vi "GEOM_GUI_trans_geom.vi"(10 "amps in":T1={"number"=0, "type"=0, "rotated"=0, "fliped"=0, "FPAcoord"={"xstart"=1, "ystart"=1}, "Physical_size"={"columns"=0, "rows"=0}, "predata"={"columns"=0, "rows"=0}, "postdata"={"columns"=0, "rows"=0}, "Req ROIs"=[], "Corr ROI"=[], "Detnumber"=0, "ampID"="", "discard"=0} {"fliped" items=["none", "horizontal", "vertical"]; "type" items=["LL", "LR", "UL", "UR"]}) -> (1 "amp direction":string, 2 "amps out":T1={"number"=0, "type"=0, "rotated"=0, "fliped"=0, "FPAcoord"={"xstart"=1, "ystart"=1}, "Physical_size"={"columns"=0, "rows"=0}, "predata"={"columns"=0, "rows"=0}, "postdata"={"columns"=0, "rows"=0}, "Req ROIs"=[], "Corr ROI"=[], "Detnumber"=0, "ampID"="", "discard"=0} {"fliped" items=["none", "horizontal", "vertical"]; "type" items=["LL", "LR", "UL", "UR"]})   [LabVIEW 2016]
uses:
  private/vis/GEOM_Amplifier.ctl
  private/vis/GEOM_AmpType.ctl
  private/vis/GEOM_ROI.ctl
  private/vis/GEOM_Coords.ctl
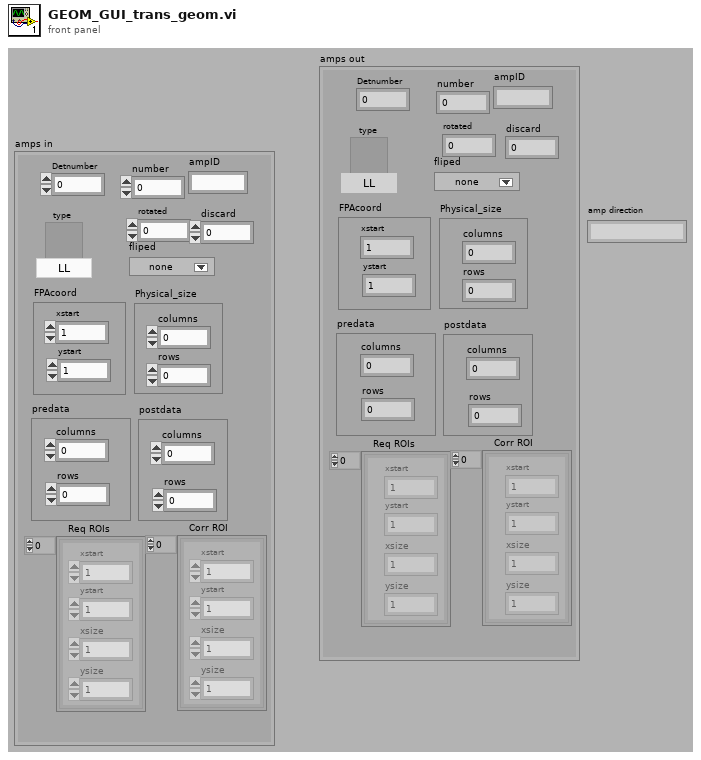
[diagram p1: front panel]
types:
  T1 = typedef "GEOM_Amplifier.ctl" = cluster{"number":i32, "type":T2, "rotated":i16, "fliped":u16, "FPAcoord":cluster{"xstart":i32, "ystart":i32}, "Physical_size":cluster{"columns":i32, "rows":i32}, "predata":cluster{"columns":i32, "rows":i32}, "postdata":cluster{"columns":i32, "rows":i32}, "Req ROIs":T3, "Corr ROI":T3, "Detnumber":i32, "ampID":string, "discard":i32}
  T2 = typedef "GEOM_AmpType.ctl" = u16
  T3 = typedef "GEOM_ROI.ctl" = T4[]
  T4 = typedef "GEOM_Coords.ctl" = cluster{"xstart":u32, "ystart":u32, "xsize":u32, "ysize":u32}
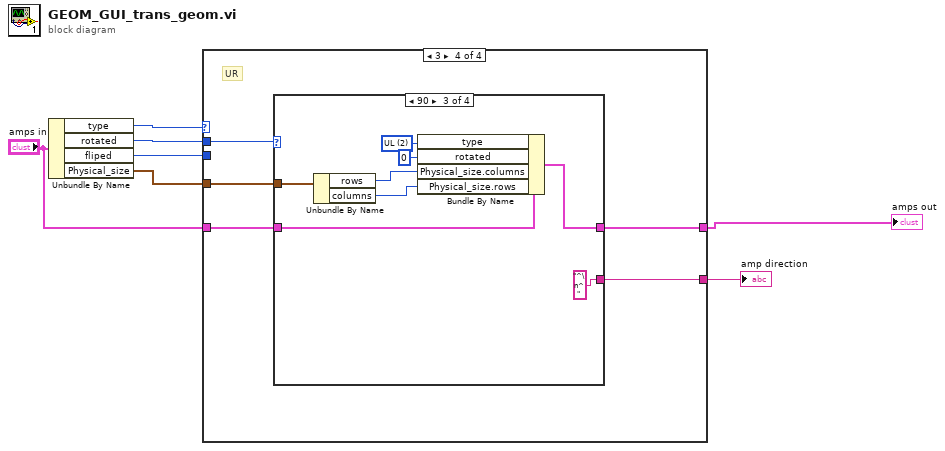
[diagram p0: block diagram]
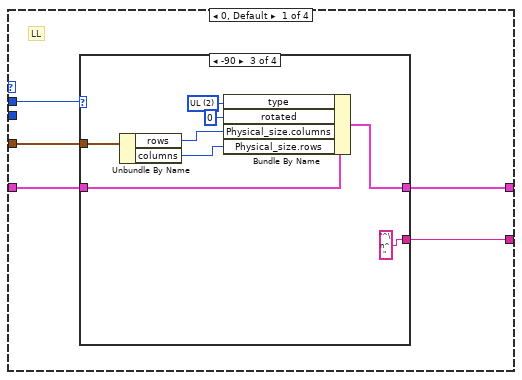
[diagram p2: hidden frame]
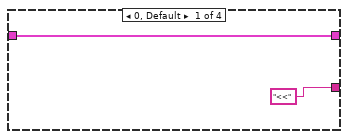
[diagram p3: hidden frame]
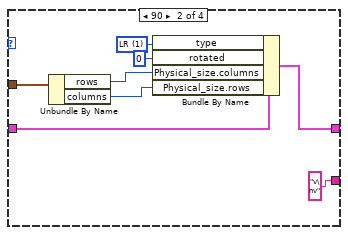
[diagram p4: hidden frame]
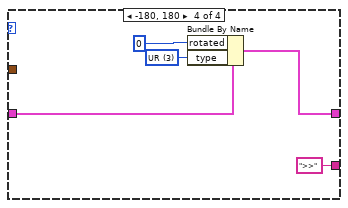
[diagram p5: hidden frame]
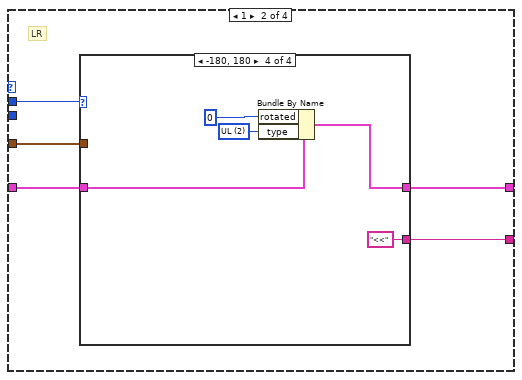
[diagram p6: hidden frame]
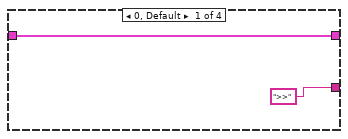
[diagram p7: hidden frame]
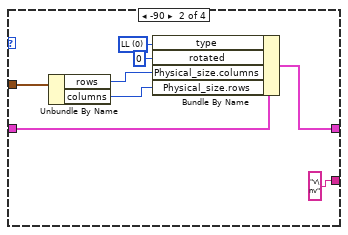
[diagram p8: hidden frame]
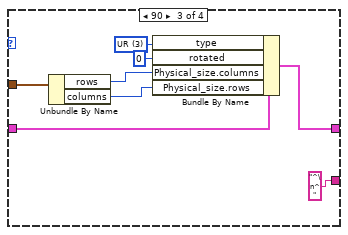
[diagram p9: hidden frame]
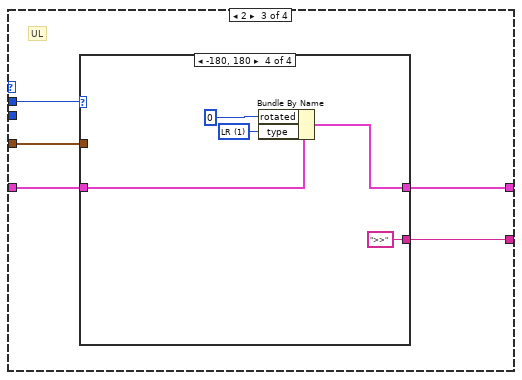
[diagram p10: hidden frame]
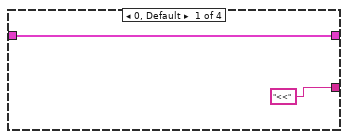
[diagram p11: hidden frame]
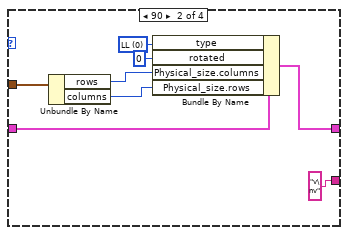
[diagram p12: hidden frame]
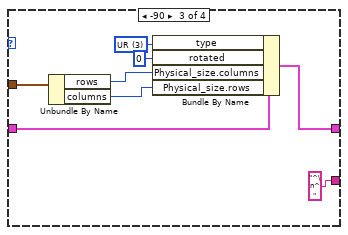
[diagram p13: hidden frame]
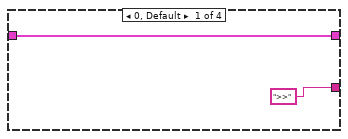
[diagram p14: hidden frame]
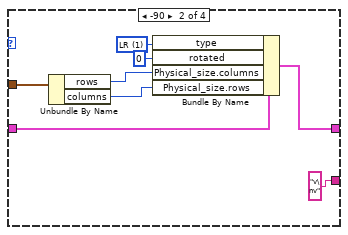
[diagram p15: hidden frame]
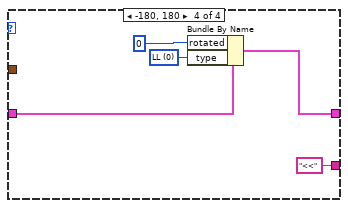
[diagram p16: hidden frame]
diagram:
  n1 = Unbundle By Name("amps in") -> ("type"=w7:T2, "rotated"=w6:i16, "fliped"=w5:u16, "Physical_size"=w4:cluster{"columns":i32, "rows":i32})
  n2 = case shown="3" w7 {
    tunnel: w6 -> [w11 w39 w67 w95]
    tunnel: w5 -> [_ _ _ _]
    tunnel: w4 -> [w12 w40 w68 w96]
    tunnel: "amps in" -> [w10 w38 w66 w94]
    tunnel: [w9 w37 w65 w93] -> w2
    tunnel: [w8 w36 w64 w92] -> w1
    frame 0, Default {
      # "LL"
      n3 = case shown="-90" w11 {
        tunnel: w10 -> [w14 w22 w30 w35]
        tunnel: [w14 w18 w26 w34] -> w9
        tunnel: w12 -> [_ w21 w29 _]
        tunnel: ["<<" "v\nv" "^\n^" ">>"] -> w8
        frame 0, Default {
        }
        frame 90 {
          w15 = T2 1 items=["LL", "LR", "UL", "UR"] ("type")
          n4 = Unbundle By Name(w21) -> ("rows"=w20:i32, "columns"=w19:i32)
          n5 = Bundle By Name(cluster=w22, "type"=w15, "rotated"=i16 0, "Physical_size.columns"=w20, "Physical_size.rows"=w19) -> (w18:T1)
        }
        frame -90 {
          w23 = T2 2 items=["LL", "LR", "UL", "UR"] ("type")
          n6 = Unbundle By Name(w29) -> ("rows"=w28:i32, "columns"=w27:i32)
          n7 = Bundle By Name(cluster=w30, "type"=w23, "rotated"=i16 0, "Physical_size.columns"=w28, "Physical_size.rows"=w27) -> (w26:T1)
        }
        frame -180, 180 {
          w31 = T2 3 items=["LL", "LR", "UL", "UR"] ("type")
          n8 = Bundle By Name(cluster=w35, "rotated"=i16 0, "type"=w31) -> (w34:T1)
        }
      }
    }
    frame 1 {
      # "LR"
      n9 = case shown="-180, 180" w39 {
        tunnel: w38 -> [w42 w50 w58 w63]
        tunnel: [w42 w46 w54 w62] -> w37
        tunnel: w40 -> [_ w49 w57 _]
        tunnel: [">>" "v\nv" "^\n^" "<<"] -> w36
        frame 0, Default {
        }
        frame -90 {
          w43 = T2 0 items=["LL", "LR", "UL", "UR"] ("type")
          n10 = Unbundle By Name(w49) -> ("rows"=w48:i32, "columns"=w47:i32)
          n11 = Bundle By Name(cluster=w50, "type"=w43, "rotated"=i16 0, "Physical_size.columns"=w48, "Physical_size.rows"=w47) -> (w46:T1)
        }
        frame 90 {
          w51 = T2 3 items=["LL", "LR", "UL", "UR"] ("type")
          n12 = Unbundle By Name(w57) -> ("rows"=w56:i32, "columns"=w55:i32)
          n13 = Bundle By Name(cluster=w58, "type"=w51, "rotated"=i16 0, "Physical_size.columns"=w56, "Physical_size.rows"=w55) -> (w54:T1)
        }
        frame -180, 180 {
          w59 = T2 2 items=["LL", "LR", "UL", "UR"] ("type")
          n14 = Bundle By Name(cluster=w63, "rotated"=i16 0, "type"=w59) -> (w62:T1)
        }
      }
    }
    frame 2 {
      # "UL"
      n15 = case shown="-180, 180" w67 {
        tunnel: w66 -> [w70 w78 w86 w91]
        tunnel: [w70 w74 w82 w90] -> w65
        tunnel: w68 -> [_ w77 w85 _]
        tunnel: ["<<" "v\nv" "^\n^" ">>"] -> w64
        frame 0, Default {
        }
        frame 90 {
          w71 = T2 0 items=["LL", "LR", "UL", "UR"] ("type")
          n16 = Unbundle By Name(w77) -> ("rows"=w76:i32, "columns"=w75:i32)
          n17 = Bundle By Name(cluster=w78, "type"=w71, "rotated"=i16 0, "Physical_size.columns"=w76, "Physical_size.rows"=w75) -> (w74:T1)
        }
        frame -90 {
          w79 = T2 3 items=["LL", "LR", "UL", "UR"] ("type")
          n18 = Unbundle By Name(w85) -> ("rows"=w84:i32, "columns"=w83:i32)
          n19 = Bundle By Name(cluster=w86, "type"=w79, "rotated"=i16 0, "Physical_size.columns"=w84, "Physical_size.rows"=w83) -> (w82:T1)
        }
        frame -180, 180 {
          w87 = T2 1 items=["LL", "LR", "UL", "UR"] ("type")
          n20 = Bundle By Name(cluster=w91, "rotated"=i16 0, "type"=w87) -> (w90:T1)
        }
      }
    }
    frame 3 {
      # "UR"
      n21 = case shown="90" w95 {
        tunnel: w94 -> [w98 w106 w114 w119]
        tunnel: [w98 w102 w110 w118] -> w93
        tunnel: w96 -> [_ w105 w113 _]
        tunnel: [">>" "v\nv" "^\n^" "<<"] -> w92
        frame 0, Default {
        }
        frame -90 {
          w99 = T2 1 items=["LL", "LR", "UL", "UR"] ("type")
          n22 = Unbundle By Name(w105) -> ("rows"=w104:i32, "columns"=w103:i32)
          n23 = Bundle By Name(cluster=w106, "type"=w99, "rotated"=i16 0, "Physical_size.columns"=w104, "Physical_size.rows"=w103) -> (w102:T1)
        }
        frame 90 {
          w107 = T2 2 items=["LL", "LR", "UL", "UR"] ("type")
          n24 = Unbundle By Name(w113) -> ("rows"=w112:i32, "columns"=w111:i32)
          n25 = Bundle By Name(cluster=w114, "type"=w107, "rotated"=i16 0, "Physical_size.columns"=w112, "Physical_size.rows"=w111) -> (w110:T1)
        }
        frame -180, 180 {
          w115 = T2 0 items=["LL", "LR", "UL", "UR"] ("type")
          n26 = Bundle By Name(cluster=w119, "rotated"=i16 0, "type"=w115) -> (w118:T1)
        }
      }
    }
  }
  "amps out" <- w2
  "amp direction" <- w1
